vi "RampPwm.vi"(10 "Ramp Step":dbl, 11 "Input":dbl) -> (3 "Output":dbl)   [LabVIEW 2014]
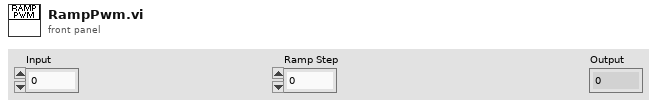
[diagram p1: front panel]
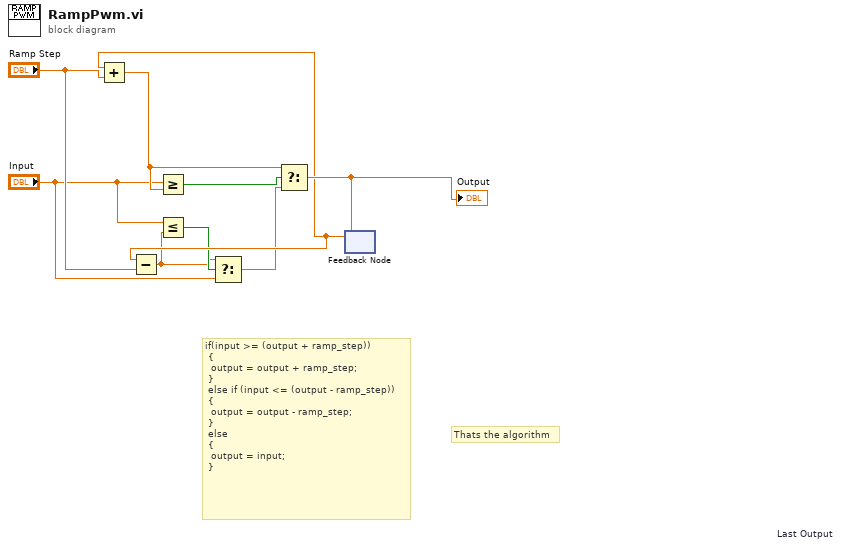
[diagram p0: block diagram]
diagram:
  # "Thats the algorithm"
  # "if(input >= (output + ramp_step))\n\t{\n\t\toutput = output + ramp_step;\n\t}\n\telse if (input <= (output - ramp_step))\n\t{\n\t\toutput = output - ramp_step;\n\t}\n\telse\n\t{\n\t\toutput = input;\n\t}"
  n1 = feedback #1 "Last Output"() -> (w6:dbl)  [unwired: 1 in]
  n2 = Add(x=w6, y="Ramp Step") -> (x+y=w7:dbl)
  n3 = Subtract(x=w6, y="Ramp Step") -> (x-y=w3:dbl)
  n4 = Greater Or Equal?(x="Input", y=w7) -> (x >= y?=w9:bool)
  n5 = Less Or Equal?(x="Input", y=w3) -> (x <= y?=w4:bool)
  n6 = Select(t=w3, s=w4, f="Input") -> (s? t:f=w1:dbl)
  n7 = Select(t=w7, s=w9, f=w1) -> (s? t:f=w8:dbl)
  "Output" <- w8
  n8 = feedback-in #1(w8) -> ()
